vi "main.vi"() -> ()   [LabVIEW 2018]
panel:
  out "开关操作":sgl[](graph)
  out "开关锁止":sgl[](graph)
  out "关开操作":sgl[](graph)
  out "关开锁止":sgl[](graph)
  out "产品名称":string
  in  "产品选择":enum32{"1", "2"}(radio)
  out "ROBOT通讯状态":bool
  out "PLC通讯状态":bool
  out "时刻":string
  in  "参数":bool
  out "F拨钮下上":string
  out "F拨钮上下":string
  out "F拨钮右左":string
  out "F拨钮左右":string
  out "F轮盘开关锁":string
  out "F轮盘开关":string
  out "F轮盘关开锁":string
  out "F轮盘关开":string
  out "LED电流":string
  out "LED电压":string
  out "风门开电压":string
  out "风门闭电压":string
  out "泄漏量结果":string
  out "压力结果":string
  out "漏装3":string
  out "漏装2":string
  out "漏装1":string
  out "风门打开标准":string
  out "风门关闭标准":string
  out "压力标准":string
  out "泄漏量标准":string
  out "LED电压标准":string
  out "LED电流标准":string
  out "拨钮左右标准":string
  out "拨钮右左标准":string
  out "拨钮上下标准":string
  out "拨钮下上标准":string
  out "轮盘关开标准":string
  out "轮盘关开锁止标准":string
  out "轮盘开关标准":string
  out "轮盘开关锁止标准":string
  in  "选项卡控件":T1(tab)
  out "海绵条":bool
  out "小齿轮":bool
  out "连杆":bool
  out "扇齿轮":bool
  out "卡扣左后":bool
  out "卡扣左前":bool
  out "卡扣右后":bool
  out "卡扣右前":bool
  out "金属4":bool
  out "金属3":bool
  out "金属2":bool
  out "金属1":bool
  out "泄漏量":sgl(knob) scale=0.0..30.0
  out "压力":sgl(knob) scale=0.0..800.0
  out "轮盘关开":sgl(graph)
  out "轮盘开关":sgl(graph)
  out "拨钮左右":sgl(graph)
  out "拨钮右左":sgl(graph)
  out "拨钮下上":sgl(graph)
  out "拨钮上下":sgl(graph)
  in  "退出":bool
  out "OK-NG":string
  # "漏装检测"
  # "泄漏检测"
  # "电检"
  # "拨钮操作力（N）"
  # "轮盘操作力矩（Ncm）"
  # "位置"
  # "结果"
  # "标准"
  # "结果"
  # "项目"
  # "标准"
  # "结果"
  # "操作方向"
  # "标准"
  # "结果"
  # "操作方向"
  # "力矩类型"
  # "标准"
  # "结果"
  # "1#位"
  # "风门打开"
  # "左->右"
  # "操作力矩"
  # "关->开"
  # "2#位"
  # "风门关闭"
  # "右->左"
  # "锁止力矩"
  # "3#位"
  # "LED电压"
  # "上->下"
  # "操作力矩"
  # "开->关"
  # "LED电流"
  # "下->上"
  # "锁止力矩"
  # "1#位"
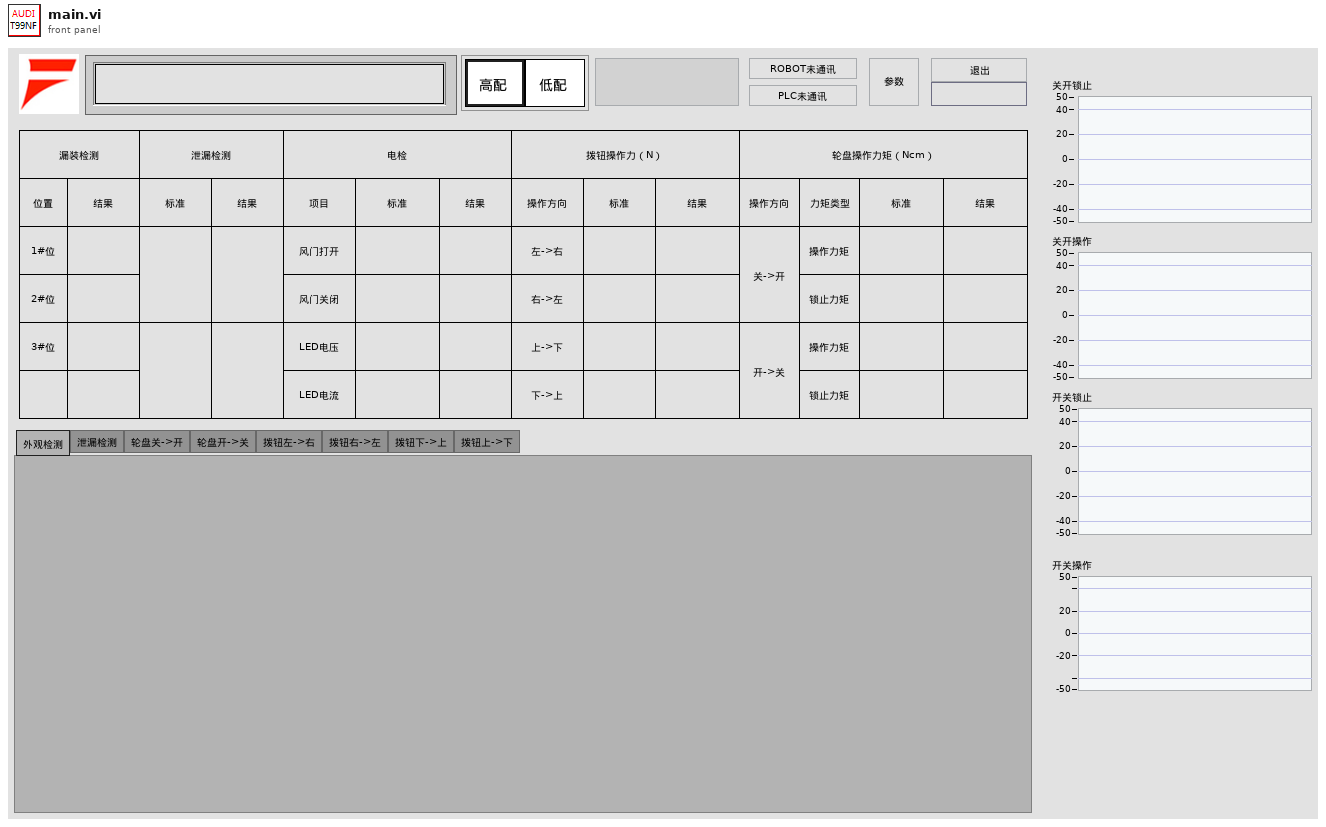
[diagram p1: front panel]
types:
  T1 = enum32{"外观检测", "泄漏检测", "轮盘关->开", "轮盘开->关", "拨钮左->右", "拨钮右->左", "拨钮下->上", "拨钮上->下"}
  T2 = cluster{"压力":string, "泄漏量":string, "风门打开":string, "风门关闭":string, "LED电压":string, "LED电流":string, "拨钮左右":string, "拨钮右左":string, "拨钮上下":string, "拨钮下上":string, "轮盘关开":string, "轮盘关开锁止":string, "轮盘开关":string, "轮盘开关锁止":string}
  T3 = enum16{"Always On", "Always Off", "Off While Running"}
  T4 = cluster{"选择":enum16{"Fx", "Fy", "Fz", "Mx", "My", "Mz"}, "系数":sgl, "上限":sgl, "下限":sgl, "Ymax":dbl, "Ymin":dbl, "点数":dbl, "锁系数x":sgl, "锁上限":sgl, "锁下限":sgl, "锁系数+":sgl, "起点":dbl, "终点":dbl, "锁起点":dbl, "锁终点":dbl}
  T5 = cluster{"选择":enum16{"Fx", "Fy", "Fz", "Mx", "My", "Mz"}, "系数":sgl, "上限":sgl, "下限":sgl, "Ymax":dbl, "Ymin":dbl, "点数":dbl, "起点":dbl, "终点":dbl}
  T6 = cluster{"PLC就绪":bool, "ROBOT就绪":bool, "空动作":bool, "检测NG":bool, "检测结束":bool, "检测开始":bool, "初始化脉冲":bool}
  T7 = cluster{"当前泄漏量":sgl, "稳定泄漏量":sgl, "当前压力":sgl, "稳定压力":sgl, "风门闭电压":sgl, "风门开电压":sgl, "LED电流":sgl, "LED电压":sgl}
  T8 = cluster{"泄漏量":bool, "风门开闭电检":bool, "LED电检":bool, "拍照位1":bool, "拍照位2":bool, "拍照位3":bool, "轮盘关开":bool, "轮盘关开锁":bool, "轮盘开关":bool, "轮盘开关锁":bool, "拨钮左右":bool, "拨钮右左":bool, "拨钮上下":bool, "拨钮下上":bool}
  T9 = cluster{"泄漏量":bool, "风门闭电压":bool, "风门开电压":bool, "LED电压":bool, "LED电流":bool, "拍照1":bool, "拍照2":bool, "拍照3":bool}
  T10 = cluster{"主站IP":u32, "组号":u8, "帧号":u16, "时间戳":u64}
  T11 = cluster{"泄漏量":bool, "轮盘开闭电检":bool, "LED电检":bool, "拍照位1":bool, "拍照位2":bool, "拍照位3":bool, "轮盘关开":bool, "轮盘关开锁":bool, "轮盘开关":bool, "轮盘开关锁":bool, "拨钮左右":bool, "拨钮右左":bool, "拨钮上下":bool, "拨钮下上":bool}
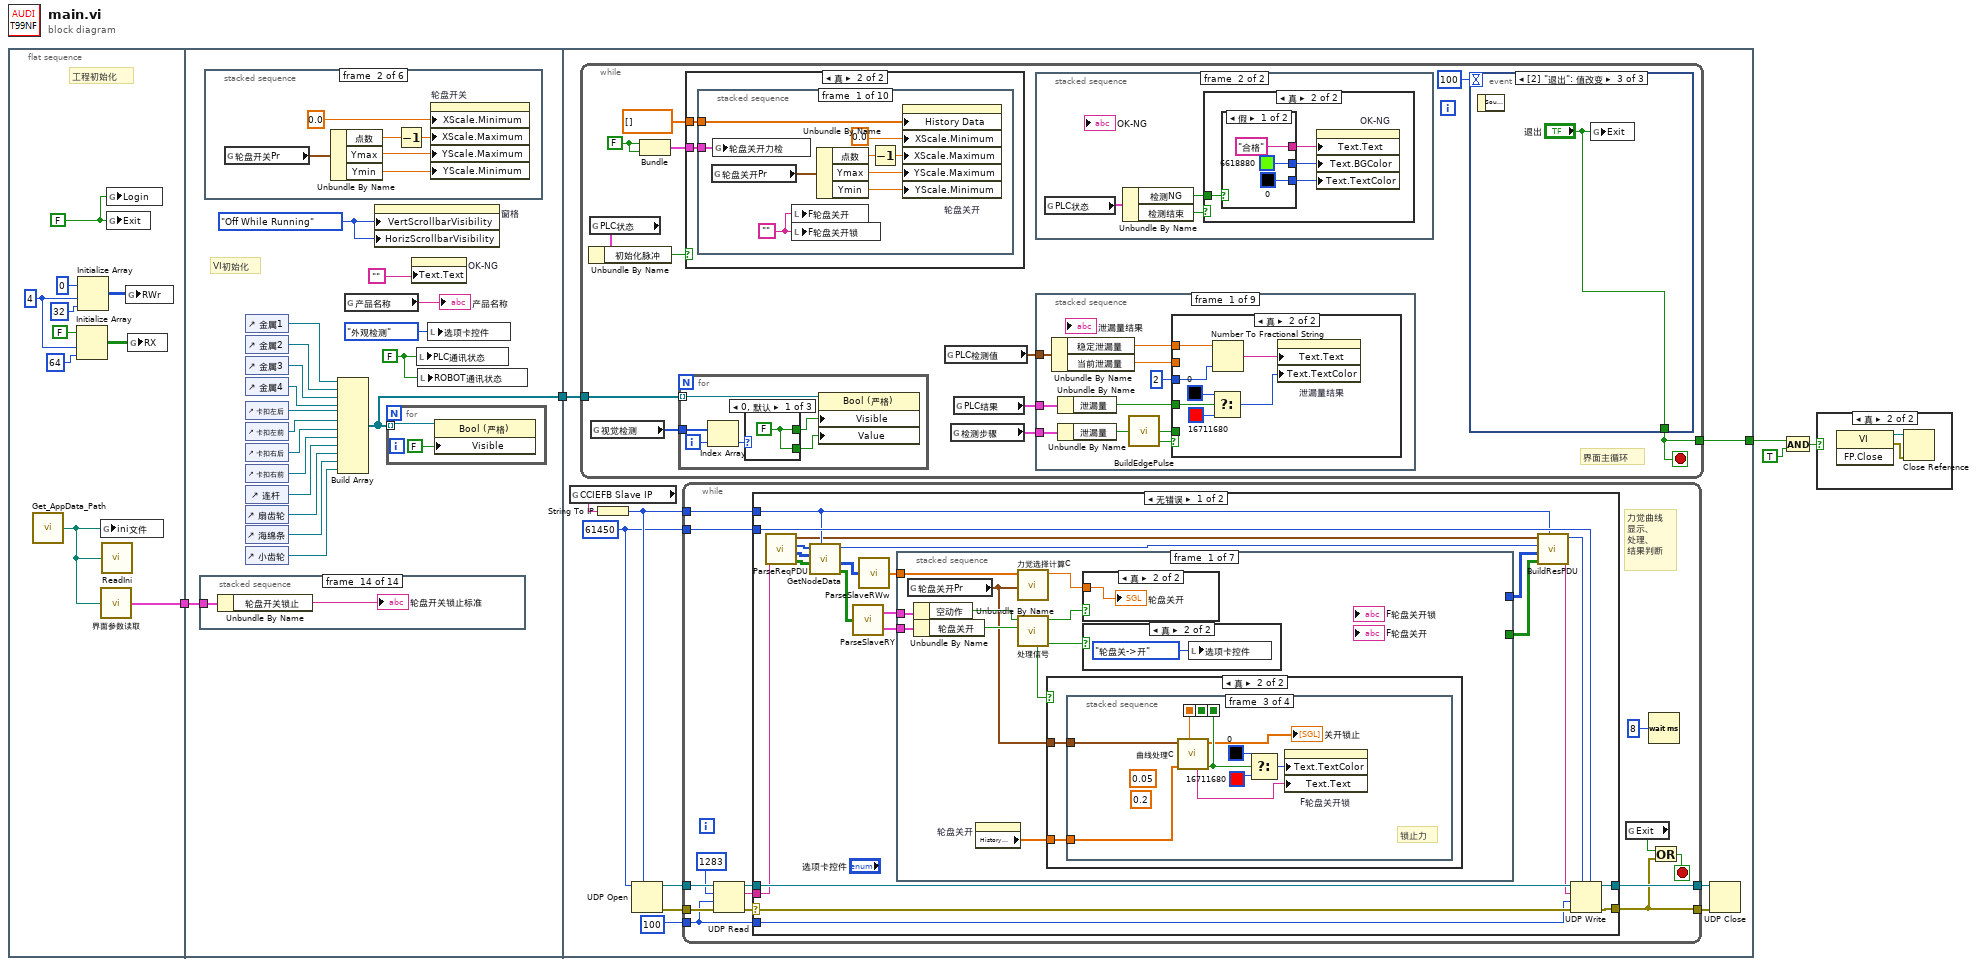
[diagram p0: block diagram]
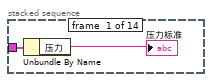
[diagram p2: hidden frame]
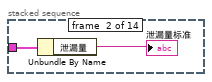
[diagram p3: hidden frame]
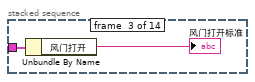
[diagram p4: hidden frame]
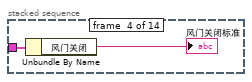
[diagram p5: hidden frame]
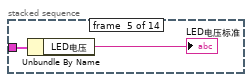
[diagram p6: hidden frame]
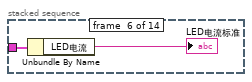
[diagram p7: hidden frame]
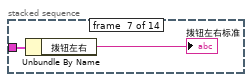
[diagram p8: hidden frame]
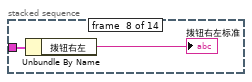
[diagram p9: hidden frame]
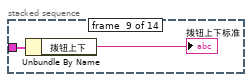
[diagram p10: hidden frame]
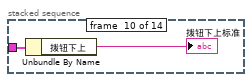
[diagram p11: hidden frame]
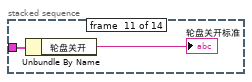
[diagram p12: hidden frame]
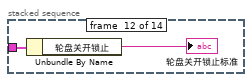
[diagram p13: hidden frame]
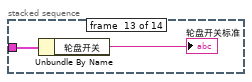
[diagram p14: hidden frame]
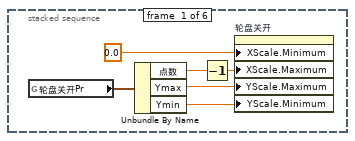
[diagram p15: hidden frame]
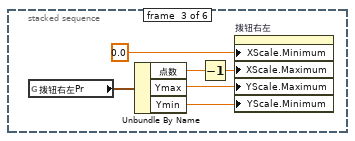
[diagram p16: hidden frame]
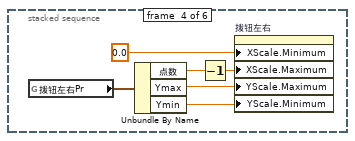
[diagram p17: hidden frame]
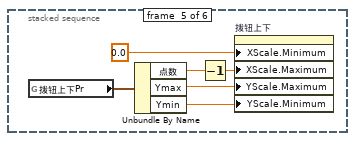
[diagram p18: hidden frame]
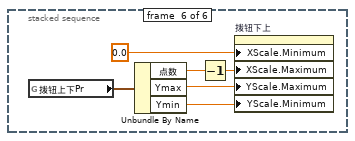
[diagram p19: hidden frame]
diagram:
  n1 = flat-sequence {
    tunnel: [w6] -> w1
    tunnel: [w21] -> w2
    tunnel: w1 -> [w16]
    tunnel: [w110] -> w4
    tunnel: w2 -> [w103]
    frame #0 {
      w11 = 4 ("维数大小")
      w8 = FALSE ("退出")
      # "工程初始化"
      n2 = call "Get_AppData_Path.vi"() -> ("path"=w7:path)  [unwired: 1 in]
      n3 = Initialize Array(FALSE, w11, 64 ("维数大小")) -> (w9:bool[][])
      n4 = Initialize Array(i16 0 ("元素"), w11, 32 ("维数大小")) -> (w14:i16[][])
      n5 = global write "全局 1.vi" "ini文件"(w7) -> ()
      n6 = call "界面参数读取.vi"("路径"=w7) -> ("标准"=w6:T2)
      n7 = call "ReadIni.vi"("configuration file path"=w7) -> ()  [unwired: 1 in]
      n8 = global write "全局 1.vi" "Login"(w8) -> ()
      n9 = global write "全局 1.vi" "Exit"(w8) -> ()
      n10 = global write "全局 1.vi" "RWr"(w14) -> ()
      n11 = global write "全局 1.vi" "RX"(w9) -> ()
    }
    frame #1 {
      w17 = T3."Off While Running" ("垂直滚动条可见")
      w18 = FALSE
      # "VI初始化"
      n12 = stacked-sequence {
        tunnel: w16 -> [w36 w38 w40 w42 w44 w46 w48 w50 w52 w54 w56 w58 w60 w62]
        frame #0 {
          n13 = Unbundle By Name(w36) -> ("压力"=→"压力标准":string)
        }
        frame #1 {
          n14 = Unbundle By Name(w38) -> ("泄漏量"=→"泄漏量标准":string)
        }
        frame #2 {
          n15 = Unbundle By Name(w40) -> ("风门打开"=→"风门打开标准":string)
        }
        frame #3 {
          n16 = Unbundle By Name(w42) -> ("风门关闭"=→"风门关闭标准":string)
        }
        frame #4 {
          n17 = Unbundle By Name(w44) -> ("LED电压"=→"LED电压标准":string)
        }
        frame #5 {
          n18 = Unbundle By Name(w46) -> ("LED电流"=→"LED电流标准":string)
        }
        frame #6 {
          n19 = Unbundle By Name(w48) -> ("拨钮左右"=→"拨钮左右标准":string)
        }
        frame #7 {
          n20 = Unbundle By Name(w50) -> ("拨钮右左"=→"拨钮右左标准":string)
        }
        frame #8 {
          n21 = Unbundle By Name(w52) -> ("拨钮上下"=→"拨钮上下标准":string)
        }
        frame #9 {
          n22 = Unbundle By Name(w54) -> ("拨钮下上"=→"拨钮下上标准":string)
        }
        frame #10 {
          n23 = Unbundle By Name(w56) -> ("轮盘关开"=→"轮盘关开标准":string)
        }
        frame #11 {
          n24 = Unbundle By Name(w58) -> ("轮盘关开锁止"=→"轮盘关开锁止标准":string)
        }
        frame #12 {
          n25 = Unbundle By Name(w60) -> ("轮盘开关"=→"轮盘开关标准":string)
        }
        frame #13 {
          n26 = Unbundle By Name(w62) -> ("轮盘开关锁止"=→"轮盘开关锁止标准":string)
        }
      }
      n27 = stacked-sequence {
        frame #0 {
          n28 = global read "全局 1.vi" "轮盘关开Pr"() -> (w68:T4)
          n29 = Unbundle By Name(w68) -> ("点数"=w64:dbl, "Ymax"=w66:dbl, "Ymin"=w67:dbl)
          n30 = Decrement(x=w64) -> (x-1=w65:dbl)
          n31 = property on="轮盘关开" class="WFChart (严格)"("XScale.Minimum"=0.0, "XScale.Maximum"=w65, "YScale.Maximum"=w66, "YScale.Minimum"=w67) -> ()  [unwired: 2 in, 2 out]
        }
        frame #1 {
          n32 = global read "全局 1.vi" "轮盘开关Pr"() -> (w74:T4)
          n33 = Unbundle By Name(w74) -> ("点数"=w70:dbl, "Ymax"=w72:dbl, "Ymin"=w73:dbl)
          n34 = Decrement(x=w70) -> (x-1=w71:dbl)
          n35 = property on="轮盘开关" class="WFChart (严格)"("XScale.Minimum"=0.0 ("X标尺.范围:最大值"), "XScale.Maximum"=w71, "YScale.Maximum"=w72, "YScale.Minimum"=w73) -> ()  [unwired: 2 in, 2 out]
        }
        frame #2 {
          n36 = global read "全局 1.vi" "拨钮右左Pr"() -> (w80:T5)
          n37 = Unbundle By Name(w80) -> ("点数"=w76:dbl, "Ymax"=w78:dbl, "Ymin"=w79:dbl)
          n38 = Decrement(x=w76) -> (x-1=w77:dbl)
          n39 = property on="拨钮右左" class="WFChart (严格)"("XScale.Minimum"=0.0 ("X标尺.范围:最大值"), "XScale.Maximum"=w77, "YScale.Maximum"=w78, "YScale.Minimum"=w79) -> ()  [unwired: 2 in, 2 out]
        }
        frame #3 {
          n40 = global read "全局 1.vi" "拨钮左右Pr"() -> (w86:T5)
          n41 = Unbundle By Name(w86) -> ("点数"=w82:dbl, "Ymax"=w84:dbl, "Ymin"=w85:dbl)
          n42 = Decrement(x=w82) -> (x-1=w83:dbl)
          n43 = property on="拨钮左右" class="WFChart (严格)"("XScale.Minimum"=0.0 ("X标尺.范围:最大值"), "XScale.Maximum"=w83, "YScale.Maximum"=w84, "YScale.Minimum"=w85) -> ()  [unwired: 2 in, 2 out]
        }
        frame #4 {
          n44 = global read "全局 1.vi" "拨钮上下Pr"() -> (w92:T5)
          n45 = Unbundle By Name(w92) -> ("点数"=w88:dbl, "Ymax"=w90:dbl, "Ymin"=w91:dbl)
          n46 = Decrement(x=w88) -> (x-1=w89:dbl)
          n47 = property on="拨钮上下" class="WFChart (严格)"("XScale.Minimum"=0.0 ("X标尺.范围:最大值"), "XScale.Maximum"=w89, "YScale.Maximum"=w90, "YScale.Minimum"=w91) -> ()  [unwired: 2 in, 2 out]
        }
        frame #5 {
          n48 = global read "全局 1.vi" "拨钮上下Pr"() -> (w98:T5)
          n49 = Unbundle By Name(w98) -> ("点数"=w94:dbl, "Ymax"=w96:dbl, "Ymin"=w97:dbl)
          n50 = Decrement(x=w94) -> (x-1=w95:dbl)
          n51 = property on="拨钮下上" class="WFChart (严格)"("XScale.Minimum"=0.0 ("X标尺.范围:最大值"), "XScale.Maximum"=w95, "YScale.Maximum"=w96, "YScale.Minimum"=w97) -> ()  [unwired: 2 in, 2 out]
        }
      }
      n52 = control-ref of="金属1"() -> (w22:refnum<vi>)
      n53 = control-ref of="金属2"() -> (w23:refnum<vi>)
      n54 = control-ref of="金属3"() -> (w24:refnum<vi>)
      n55 = control-ref of="金属4"() -> (w25:refnum<vi>)
      n56 = control-ref of="卡扣左后"() -> (w26:refnum<vi>)
      n57 = control-ref of="卡扣左前"() -> (w27:refnum<vi>)
      n58 = control-ref of="卡扣右后"() -> (w28:refnum<vi>)
      n59 = control-ref of="卡扣右前"() -> (w29:refnum<vi>)
      n60 = control-ref of="连杆"() -> (w30:refnum<vi>)
      n61 = control-ref of="扇齿轮"() -> (w31:refnum<vi>)
      n62 = control-ref of="海绵条"() -> (w32:refnum<vi>)
      n63 = control-ref of="小齿轮"() -> (w33:refnum<vi>)
      n64 = Build Array(w22, w23, w24, w25, w26, w27, w28, w29, w30, w31, w32, w33) -> (w21:refnum<vi>[])
      n65 = global read "全局 1.vi" "产品名称"() -> (→"产品名称":string)
      n66 = property on="窗格" class="Pane"("VertScrollbarVisibility"=w17, "HorizScrollbarVisibility"=w17) -> ()  [unwired: 2 in, 2 out]
      n67 = for {
        tunnel: w21 -> [w100] mode=indexing
        n68 = property class="Bool (严格)"(reference=w100, "Visible"=FALSE ("可见")) -> ()  [unwired: 1 in, 2 out]
      }
      n69 = property on="OK-NG" class="Str"("Text.Text"="") -> ()  [unwired: 2 in, 2 out]
      n70 = local write "PLC通讯状态"(w18) -> ()
      n71 = local write "ROBOT通讯状态"(w18) -> ()
      n72 = local write "选项卡控件"(T1."外观检测" ("选项卡控件")) -> ()
    }
    frame #2 {
      w104 = u16 61450 ("端口")
      n73 = global read "全局 1.vi" "CCIEFB Slave IP"() -> (w102:string)
      n74 = while {
        tunnel: [w409] -> w110
        tunnel: w103 -> [w407]
        stop <- w409 stop-if-true
        w406 = FALSE
        # "界面主循环"
        n75 = global read "全局 1.vi" "PLC状态"() -> (w404:T6)
        n76 = Unbundle By Name(w404) -> ("初始化脉冲"=w403:bool)
        n77 = global read "全局 1.vi" "视觉检测"() -> (w408:u16[])
        n78 = Bundle(w406, w406) -> (w405:cluster{bool, bool})  [unwired: 1 in]
        n79 = for {
          tunnel: w407 -> [w652] mode=indexing
          tunnel: w408 -> [w655]
          i -> [w654]
          n80 = Index Array(array=w655, index=w654) -> (element=w653:u16)
          n81 = case shown="0, 默认" w653 {
            tunnel: [w656 TRUE TRUE] -> w651
            tunnel: [w656 FALSE TRUE] -> w650
            frame 0, Default {
              w656 = FALSE
            }
            frame 1 {
            }
            frame 2 {
            }
          }
          n82 = property class="Bool (严格)"(reference=w652, "Visible"=w651, "Value"=w650) -> ()  [unwired: 1 in, 2 out]
        }
        n83 = case shown="真" w403 {
          tunnel: w405 -> [_ w590]
          tunnel: sgl[] [] ("历史数据") -> [_ w589]
          frame False {
          }
          frame True {
            n84 = stacked-sequence {
              tunnel: w590 -> [w599 _ w609 _ w619 w628 w637 w646 _ _]
              tunnel: w589 -> [w591 w600 w601 w610 w611 w620 w629 w638 _ _]
              frame #0 {
                w592 = ""
                n85 = global read "全局 1.vi" "轮盘关开Pr"() -> (w597:T4)
                n86 = global write "全局 1.vi" "轮盘关开力检"(w599) -> ()
                n87 = local write "F轮盘关开"(w592) -> ()
                n88 = local write "F轮盘关开锁"(w592) -> ()
                n89 = Unbundle By Name(w597) -> ("点数"=w598:dbl, "Ymax"=w594:dbl, "Ymin"=w593:dbl)
                n90 = Decrement(x=w598) -> (x-1=w596:dbl)
                n91 = property on="轮盘关开" class="WFChart (严格)"("History Data"=w591, "XScale.Minimum"=0.0, "XScale.Maximum"=w596, "YScale.Maximum"=w594, "YScale.Minimum"=w593) -> ()  [unwired: 2 in, 2 out]
              }
              frame #1 {
                n92 = property on="关开锁止" class="WFChart (严格)"("History Data"=w600) -> ()  [unwired: 2 in, 2 out]
                n93 = property on="关开操作" class="WFChart (严格)"("History Data"=w600) -> ()  [unwired: 2 in, 2 out]
              }
              frame #2 {
                w602 = ""
                n94 = global write "全局 1.vi" "轮盘开关力检"(w609) -> ()
                n95 = global read "全局 1.vi" "轮盘开关Pr"() -> (w608:T4)
                n96 = local write "F轮盘开关"(w602) -> ()
                n97 = local write "F轮盘开关锁"(w602) -> ()
                n98 = Unbundle By Name(w608) -> ("点数"=w607:dbl, "Ymax"=w606:dbl, "Ymin"=w605:dbl)
                n99 = Decrement(x=w607) -> (x-1=w604:dbl)
                n100 = property on="轮盘开关" class="WFChart (严格)"("History Data"=w601, "XScale.Minimum"=0.0 ("X标尺.范围:最大值"), "XScale.Maximum"=w604, "YScale.Maximum"=w606, "YScale.Minimum"=w605) -> ()  [unwired: 2 in, 2 out]
              }
              frame #3 {
                n101 = property on="开关锁止" class="WFChart (严格)"("History Data"=w610) -> ()  [unwired: 2 in, 2 out]
                n102 = property on="开关操作" class="WFChart (严格)"("History Data"=w610) -> ()  [unwired: 2 in, 2 out]
              }
              frame #4 {
                n103 = global write "全局 1.vi" "拨钮右左力检"(w619) -> ()
                n104 = global read "全局 1.vi" "拨钮右左Pr"() -> (w618:T5)
                n105 = local write "F拨钮左右"("") -> ()
                n106 = Unbundle By Name(w618) -> ("点数"=w617:dbl, "Ymax"=w614:dbl, "Ymin"=w613:dbl)
                n107 = Decrement(x=w617) -> (x-1=w616:dbl)
                n108 = property on="拨钮右左" class="WFChart (严格)"("History Data"=w611, "XScale.Minimum"=0.0 ("X标尺.范围:最大值"), "XScale.Maximum"=w616, "YScale.Maximum"=w614, "YScale.Minimum"=w613) -> ()  [unwired: 2 in, 2 out]
              }
              frame #5 {
                n109 = global read "全局 1.vi" "拨钮左右Pr"() -> (w627:T5)
                n110 = global write "全局 1.vi" "拨钮左右力检"(w628) -> ()
                n111 = local write "F拨钮右左"("") -> ()
                n112 = Unbundle By Name(w627) -> ("点数"=w626:dbl, "Ymax"=w623:dbl, "Ymin"=w622:dbl)
                n113 = Decrement(x=w626) -> (x-1=w625:dbl)
                n114 = property on="拨钮左右" class="WFChart (严格)"("History Data"=w620, "XScale.Minimum"=0.0 ("X标尺.范围:最大值"), "XScale.Maximum"=w625, "YScale.Maximum"=w623, "YScale.Minimum"=w622) -> ()  [unwired: 2 in, 2 out]
              }
              frame #6 {
                n115 = global read "全局 1.vi" "拨钮上下Pr"() -> (w636:T5)
                n116 = global write "全局 1.vi" "拨钮下上力检"(w637) -> ()
                n117 = local write "F拨钮上下"("") -> ()
                n118 = Unbundle By Name(w636) -> ("点数"=w635:dbl, "Ymax"=w632:dbl, "Ymin"=w631:dbl)
                n119 = Decrement(x=w635) -> (x-1=w634:dbl)
                n120 = property on="拨钮下上" class="WFChart (严格)"("History Data"=w629, "XScale.Minimum"=0.0 ("X标尺.范围:最大值"), "XScale.Maximum"=w634, "YScale.Maximum"=w632, "YScale.Minimum"=w631) -> ()  [unwired: 2 in, 2 out]
              }
              frame #7 {
                n121 = global write "全局 1.vi" "拨钮上下力检"(w646) -> ()
                n122 = global read "全局 1.vi" "拨钮下上Pr"() -> (w645:T5)
                n123 = local write "F拨钮下上"("") -> ()
                n124 = Unbundle By Name(w645) -> ("点数"=w644:dbl, "Ymax"=w641:dbl, "Ymin"=w640:dbl)
                n125 = Decrement(x=w644) -> (x-1=w643:dbl)
                n126 = property on="拨钮上下" class="WFChart (严格)"("History Data"=w638, "XScale.Minimum"=0.0 ("X标尺.范围:最大值"), "XScale.Maximum"=w643, "YScale.Maximum"=w641, "YScale.Minimum"=w640) -> ()  [unwired: 2 in, 2 out]
              }
              frame #8 {
                w647 = ""
                n127 = local write "泄漏量结果"(w647) -> ()
                n128 = local write "风门开电压"(w647) -> ()
                n129 = local write "风门闭电压"(w647) -> ()
                n130 = local write "压力结果"(w647) -> ()
                n131 = local write "LED电压"(w647) -> ()
                n132 = local write "LED电流"(w647) -> ()
                n133 = local write "漏装1"(w647) -> ()
                n134 = local write "漏装2"(w647) -> ()
                n135 = local write "漏装3"(w647) -> ()
              }
              frame #9 {
                n136 = property on="OK-NG" class="Str"("Text.Text"="", "Text.BGColor"=u32 14869218) -> ()  [unwired: 2 in, 2 out]
              }
            }
          }
        }
        n137 = global read "全局 1.vi" "PLC检测值"() -> (w401:T7)
        n138 = global read "全局 1.vi" "检测步骤"() -> (w402:T8)
        n139 = global read "全局 1.vi" "PLC结果"() -> (w400:T9)
        n140 = stacked-sequence {
          frame #0 {
            n141 = global read "全局 1.vi" "PC状态"() -> (w567:cluster{"PLC就绪":bool, "空动作中":bool})
            n142 = Bundle By Name(cluster=w567, "PLC就绪"=TRUE) -> (w565:cluster{"PLC就绪":bool, "空动作中":bool})
            n143 = global read "全局 1.vi" "PLC状态"() -> (w568:T6)
            n144 = To Word Integer(number="产品选择") -> (16bit integer=w575:i16)
            n145 = Format Date/Time String(time format string (%c)="%c\n第%W周 %A" ("时间格式字符串(%c)")) -> (date/time string=→"时刻":string)  [unwired: 2 in]
            n146 = Increment(x=w575) -> (x+1=w573:i16)
            n147 = Unbundle By Name(w568) -> ("PLC就绪"=→"PLC通讯状态":bool, "ROBOT就绪"=→"ROBOT通讯状态":bool)
            n148 = global write "全局 1.vi" "PC状态"(w565) -> ()
            n149 = global write "全局 1.vi" "高低配"(w573) -> ()
          }
          frame #1 {
            n150 = global read "全局 1.vi" "PLC状态"() -> (w578:T6)
            n151 = Unbundle By Name(w578) -> ("检测NG"=w576:bool, "检测结束"=w577:bool)
            n152 = case shown="真" w577 {
              tunnel: w576 -> [_ w582]
              frame False {
              }
              frame True {
                n153 = case shown="假" w582 {
                  tunnel: ["合格" "不合格"] -> w581
                  tunnel: [u32 6618880 u32 16711680] -> w580
                  tunnel: [u32 0 u32 16448250] -> w579
                  frame False {
                  }
                  frame True {
                  }
                }
                n154 = property on="OK-NG" class="Str"("Text.Text"=w581, "Text.BGColor"=w580, "Text.TextColor"=w579) -> ()  [unwired: 2 in, 2 out]
              }
            }
          }
        }
        n155 = stacked-sequence {
          tunnel: w402 -> [w420 w444 w467 w483 w499 w515 w527 w541 w555]
          tunnel: w401 -> [w417 w441 w464 w480 w496 w512 _ _ _]
          tunnel: w400 -> [w413 w437 w461 w477 w493 w509 w524 w538 w552]
          frame #0 {
            n156 = Unbundle By Name(w417) -> ("稳定泄漏量"=w415:sgl, "当前泄漏量"=w416:sgl)
            n157 = Unbundle By Name(w413) -> ("泄漏量"=w412:bool)
            n158 = Unbundle By Name(w420) -> ("泄漏量"=w419:bool)
            n159 = call "BuildEdgePulse.vi"("输入"=w419) -> ("下降沿"=w418:bool, "输出"=w414:bool)  [unwired: 2 in, 1 out]
            n160 = case shown="真" w418 {
              tunnel: w416 -> [w423 _]
              tunnel: w415 -> [_ w433]
              tunnel: w414 -> [w422 _]
              tunnel: w412 -> [_ w432]
              tunnel: i16 2 ("精度(6)") -> [w421 w428]
              frame False {
                n161 = case shown="真" w422 {
                  tunnel: w423 -> [_ w425]
                  tunnel: w421 -> [_ w424]
                  frame False {
                  }
                  frame True {
                    n162 = Number To Fractional String(number=w425, precision (6)=w424) -> (F-format string=w427:string)  [unwired: 2 in]
                    n163 = property on="泄漏量结果" class="Str"("Text.Text"=w427, "Text.TextColor"=u32 0) -> ()  [unwired: 2 in, 2 out]
                    "泄漏量" <- w425
                  }
                }
              }
              frame True {
                n164 = Select(t=u32 0, s=w432, f=u32 16711680) -> (s? t:f=w429:u32)
                n165 = Number To Fractional String(number=w433, precision (6)=w428) -> (F-format string=w434:string)  [unwired: 2 in]
                n166 = property on="泄漏量结果" class="Str"("Text.Text"=w434, "Text.TextColor"=w429) -> ()  [unwired: 2 in, 2 out]
              }
            }
          }
          frame #1 {
            n167 = Unbundle By Name(w441) -> ("稳定压力"=w439:sgl, "当前压力"=w440:sgl)
            n168 = Unbundle By Name(w437) -> ("泄漏量"=w436:bool)
            n169 = Unbundle By Name(w444) -> ("泄漏量"=w443:bool)
            n170 = call "BuildEdgePulse.vi"("输入"=w443) -> ("下降沿"=w442:bool, "输出"=w438:bool)  [unwired: 2 in, 1 out]
            n171 = case shown="假" w442 {
              tunnel: w440 -> [w447 _]
              tunnel: w439 -> [_ w457]
              tunnel: w438 -> [w446 _]
              tunnel: w436 -> [_ w456]
              tunnel: i16 1 ("精度(6)") -> [w445 w452]
              frame False {
                n172 = case shown="真" w446 {
                  tunnel: w447 -> [_ w449]
                  tunnel: w445 -> [_ w448]
                  frame False {
                  }
                  frame True {
                    n173 = Number To Fractional String(number=w449, precision (6)=w448) -> (F-format string=w451:string)  [unwired: 2 in]
                    n174 = property on="压力结果" class="Str"("Text.Text"=w451, "Text.TextColor"=u32 0) -> ()  [unwired: 2 in, 2 out]
                    "压力" <- w449
                  }
                }
              }
              frame True {
                n175 = Select(t=u32 0, s=w456, f=u32 16711680) -> (s? t:f=w453:u32)
                n176 = Number To Fractional String(number=w457, precision (6)=w452) -> (F-format string=w458:string)  [unwired: 2 in]
                n177 = property on="压力结果" class="Str"("Text.Text"=w458, "Text.TextColor"=w453) -> ()  [unwired: 2 in, 2 out]
              }
            }
          }
          frame #2 {
            n178 = Unbundle By Name(w467) -> ("风门开闭电检"=w466:bool)
            n179 = Unbundle By Name(w461) -> ("风门开电压"=w460:bool)
            n180 = Unbundle By Name(w464) -> ("风门开电压"=w463:sgl)
            n181 = call "BuildEdgePulse.vi"("输入"=w466) -> ("下降沿"=w465:bool, "输出"=w462:bool)  [unwired: 2 in, 1 out]
            n182 = case shown="真" w465 {
              tunnel: w463 -> [_ w474]
              tunnel: w462 -> [_ _]
              tunnel: w460 -> [_ w473]
              tunnel: i16 2 ("精度(6)") -> [_ w469]
              frame False {
              }
              frame True {
                n183 = Number To Fractional String(number=w474, precision (6)=w469) -> (F-format string=→"风门开电压":string)  [unwired: 2 in]
                n184 = Select(t=u32 0, s=w473, f=u32 16711680) -> (s? t:f=w470:u32)
                n185 = property on="风门开电压" class="Str"("Text.TextColor"=w470) -> ()  [unwired: 2 in, 2 out]
              }
            }
          }
          frame #3 {
            n186 = Unbundle By Name(w483) -> ("风门开闭电检"=w482:bool)
            n187 = Unbundle By Name(w477) -> ("风门闭电压"=w476:bool)
            n188 = Unbundle By Name(w480) -> ("风门闭电压"=w479:sgl)
            n189 = call "BuildEdgePulse.vi"("输入"=w482) -> ("下降沿"=w481:bool, "输出"=w478:bool)  [unwired: 2 in, 1 out]
            n190 = case shown="真" w481 {
              tunnel: w479 -> [_ w490]
              tunnel: w478 -> [_ _]
              tunnel: w476 -> [_ w489]
              tunnel: i16 2 ("精度(6)") -> [_ w485]
              frame False {
              }
              frame True {
                n191 = Number To Fractional String(number=w490, precision (6)=w485) -> (F-format string=→"风门闭电压":string)  [unwired: 2 in]
                n192 = Select(t=u32 0, s=w489, f=u32 16711680) -> (s? t:f=w486:u32)
                n193 = property on="风门闭电压" class="Str"("Text.TextColor"=w486) -> ()  [unwired: 2 in, 2 out]
              }
            }
          }
          frame #4 {
            n194 = Unbundle By Name(w493) -> ("LED电压"=w492:bool)
            n195 = Unbundle By Name(w499) -> ("LED电检"=w498:bool)
            n196 = Unbundle By Name(w496) -> ("LED电压"=w495:sgl)
            n197 = call "BuildEdgePulse.vi"("输入"=w498) -> ("下降沿"=w497:bool, "输出"=w494:bool)  [unwired: 2 in, 1 out]
            n198 = case shown="真" w497 {
              tunnel: w495 -> [_ w506]
              tunnel: w494 -> [_ _]
              tunnel: w492 -> [_ w505]
              tunnel: i16 2 ("精度(6)") -> [_ w501]
              frame False {
              }
              frame True {
                n199 = Number To Fractional String(number=w506, precision (6)=w501) -> (F-format string=→"LED电压":string)  [unwired: 2 in]
                n200 = Select(t=u32 0, s=w505, f=u32 16711680) -> (s? t:f=w502:u32)
                n201 = property on="LED电压" class="Str"("Text.TextColor"=w502) -> ()  [unwired: 2 in, 2 out]
              }
            }
          }
          frame #5 {
            n202 = Unbundle By Name(w509) -> ("LED电流"=w508:bool)
            n203 = Unbundle By Name(w515) -> ("LED电检"=w514:bool)
            n204 = Unbundle By Name(w512) -> ("LED电流"=w511:sgl)
            n205 = call "BuildEdgePulse.vi"("输入"=w514) -> ("下降沿"=w513:bool, "输出"=w510:bool)  [unwired: 2 in, 1 out]
            n206 = case shown="真" w513 {
              tunnel: w511 -> [_ w522]
              tunnel: w510 -> [_ _]
              tunnel: w508 -> [_ w521]
              tunnel: i16 2 ("精度(6)") -> [_ w517]
              frame False {
              }
              frame True {
                n207 = Number To Fractional String(number=w522, precision (6)=w517) -> (F-format string=→"LED电流":string)  [unwired: 2 in]
                n208 = Select(t=u32 0, s=w521, f=u32 16711680) -> (s? t:f=w518:u32)
                n209 = property on="LED电流" class="Str"("Text.TextColor"=w518) -> ()  [unwired: 2 in, 2 out]
              }
            }
          }
          frame #6 {
            n210 = Unbundle By Name(w527) -> ("拍照位1"=w526:bool)
            n211 = Unbundle By Name(w524) -> ("拍照1"=w523:bool)
            n212 = call "BuildEdgePulse.vi"("输入"=w526) -> ("下降沿"=w525:bool, "上升沿"=w528:bool)  [unwired: 2 in, 1 out]
            n213 = case shown="真" w528 {
              frame False {
              }
              frame True {
                n214 = local write "选项卡控件"(T1."外观检测" ("选项卡控件")) -> ()
              }
            }
            n215 = case shown="真" w525 {
              tunnel: w523 -> [_ w531]
              frame False {
              }
              frame True {
                n216 = case shown="假" w531 {
                  tunnel: ["NG" ("文本.文本") "OK" ("文本.文本")] -> w530
                  tunnel: [u32 16711680 u32 0] -> w529
                  frame False {
                  }
                  frame True {
                  }
                }
                n217 = property on="漏装1" class="Str"("Text.Text"=w530, "Text.TextColor"=w529) -> ()  [unwired: 2 in, 2 out]
              }
            }
          }
          frame #7 {
            n218 = Unbundle By Name(w541) -> ("拍照位2"=w540:bool)
            n219 = Unbundle By Name(w538) -> ("拍照2"=w537:bool)
            n220 = call "BuildEdgePulse.vi"("输入"=w540) -> ("下降沿"=w539:bool, "上升沿"=w542:bool)  [unwired: 2 in, 1 out]
            n221 = case shown="真" w542 {
              frame False {
              }
              frame True {
                n222 = local write "选项卡控件"(T1."外观检测" ("选项卡控件")) -> ()
              }
            }
            n223 = case shown="真" w539 {
              tunnel: w537 -> [_ w545]
              frame False {
              }
              frame True {
                n224 = case shown="假" w545 {
                  tunnel: ["NG" ("文本.文本") "OK" ("文本.文本")] -> w544
                  tunnel: [u32 16711680 u32 0] -> w543
                  frame False {
                  }
                  frame True {
                  }
                }
                n225 = property on="漏装2" class="Str"("Text.Text"=w544, "Text.TextColor"=w543) -> ()  [unwired: 2 in, 2 out]
              }
            }
          }
          frame #8 {
            n226 = Unbundle By Name(w555) -> ("拍照位3"=w554:bool)
            n227 = Unbundle By Name(w552) -> ("拍照3"=w551:bool)
            n228 = call "BuildEdgePulse.vi"("输入"=w554) -> ("下降沿"=w553:bool, "上升沿"=w556:bool)  [unwired: 2 in, 1 out]
            n229 = case shown="真" w556 {
              frame False {
              }
              frame True {
                n230 = local write "选项卡控件"(T1."外观检测" ("选项卡控件")) -> ()
              }
            }
            n231 = case shown="真" w553 {
              tunnel: w551 -> [_ w559]
              frame False {
              }
              frame True {
                n232 = case shown="假" w559 {
                  tunnel: ["NG" ("文本.文本") "OK" ("文本.文本")] -> w558
                  tunnel: [u32 16711680 u32 0] -> w557
                  frame False {
                  }
                  frame True {
                  }
                }
                n233 = property on="漏装3" class="Str"("Text.Text"=w558, "Text.TextColor"=w557) -> ()  [unwired: 2 in, 2 out]
              }
            }
          }
        }
        n234 = event shown="[2] \"退出\": 值改变" {
          selector: _ -> [_ _ _]
          dyn-events: _ -> [_ _ _]
          timeout: 100 ("等待时间（毫秒）") -> [_ _ _]
          tunnel: [_ _ "退出"] -> w409
          event Timeout {
            n235 = event-data() -> ()  [unwired: 1 in, 1 out]
          }
          event "参数": Mouse Up {
            w664 = FALSE ("结束前等待")
            n236 = event-data() -> ()  [unwired: 1 in, 1 out]
            n237 = vi-ref "参数.vi"() -> (w665:refnum<vi>)
            n238 = invoke class="VI" method="Run VI"(reference=w665, "Wait until done"=w664, "Auto Dispose Ref"=w664) -> (reference out=w663:refnum<vi>)  [unwired: 2 in, 4 out]
            n239 = invoke class="VI" method="FP.Open"(reference=w663) -> (reference out=w661:refnum<vi>, error out=w662:errorcluster)  [unwired: 4 in, 3 out]
            n240 = Close Reference(reference=w661, error in (no error)=w662) -> ()  [unwired: 1 out]
          }
          event "退出": Value Change {
            n241 = event-data() -> ()  [unwired: 1 in, 1 out]
            n242 = global write "全局 1.vi" "Exit"("退出") -> ()
          }
        }
      }
      n243 = String To IP(1:w102) -> (0:w105:u32)
      n244 = UDP Open(7:w105, 11:w104) -> (port=w109:refnum<k16>, 0:w107:errorcluster)  [unwired: 3 in, 1 out]
      n245 = while {
        tunnel: w109 -> [w124]
        tunnel: [w115] -> w108
        tunnel: w107 -> [w123]
        tunnel: [w113] -> w106
        tunnel: w105 -> [w117]
        tunnel: w104 -> [w116]
        tunnel: 100 ("超时毫秒(25000)") -> [w111]
        stop <- w120 stop-if-true
        # "力觉曲线\n显示、\n处理、\n结果判断"
        n246 = UDP Read(connection ID=w124, max size (548)=1283 ("最大值(548)"), timeout ms (25000)=w111, 8:w123) -> (data out=w121:string, error out=w122:errorcluster, 3:w118:refnum<k16>)  [unwired: 2 out]
        n247 = case shown="无错误" w122 {
          selector: w122 -> [w146 w395]
          tunnel: w121 -> [w141 _]
          tunnel: [w145 w394] -> w113
          tunnel: w118 -> [w144 w393]
          tunnel: w117 -> [w138 _]
          tunnel: w116 -> [w142 _]
          tunnel: [w143 w393] -> w115
          tunnel: w111 -> [w133 _]
          frame No Error {
            n248 = call "ParseReqPDU.vi"("数据in"=w141) -> ("All RY"=w134:bool[][], "All RWw"=w135:u16[][], "从站IP组"=w137:u32[], "主站信息"=w132:T10)  [unwired: 7 in]
            n249 = call "GetNodeData.vi"("指定从站IP"=w138, "All RY in"=w134, "All RWw in"=w135, "从站IP组"=w137) -> ("Node RY"=w129:bool[][], "Node RWw"=w130:u16[][], "占用站数"=w136:i32)  [unwired: 5 in]
            n250 = call "ParseSlaveRY.vi"("RY"=w129) -> ("PLC状态"=w128:T6, "检测步骤"=w127:T11)
            n251 = call "ParseSlaveRWw.vi"("Node RWw"=w130) -> ("力觉力"=w131:sgl[])
            n252 = stacked-sequence {
              tunnel: w131 -> [w155 w203 w253 w290 w327 w364 _]
              tunnel: w128 -> [w157 w205 w252 w289 w326 w363 _]
              tunnel: w127 -> [w156 w204 w251 w288 w325 w362 _]
              tunnel: [_ _ _ _ _ _ w392] -> w126
              tunnel: [_ _ _ _ _ _ w391] -> w125
              frame #0 {
                n253 = global read "全局 1.vi" "轮盘关开Pr"() -> (w147:T4)
                n254 = Unbundle By Name(w157) -> ("空动作"=w152:bool)
                n255 = Unbundle By Name(w156) -> ("轮盘关开"=w153:bool)
                n256 = property on="轮盘关开" class="WFChart (严格)"() -> ("History Data"=w154:sgl[])  [unwired: 2 in, 2 out]
                n257 = call "力觉选择计算C.vi"("力参数C"=w147, "力"=w155) -> ("曲线"=w150:sgl)  [unwired: 8 in, 1 out]
                n258 = call "处理信号.vi"("动作"=w153, "空动作"=w152) -> ("切换"=w149:bool, "显示曲线"=w151:bool, "判断"=w148:bool)  [unwired: 7 in]
                n259 = case shown="真" w148 {
                  tunnel: w147 -> [_ w161]
                  tunnel: w154 -> [_ w160]
                  frame False {
                  }
                  frame True {
                    n260 = stacked-sequence {
                      seq-local: [_ w175 _ _] -> [_ _ _ w189]
                      seq-local: [_ w167 _ _] -> [_ _ w185 _]
                      seq-local: [_ _ w183 _] -> [_ _ _ w190]
                      tunnel: w161 -> [_ w173 w181 _]
                      tunnel: w160 -> [w162 w174 w180 _]
                      frame #0 {
                        # "显示曲线"
                        n261 = Array Size(array=w162) -> (size(s)=w165:i32)
                        n262 = Decrement(x=w165) -> (x-1=w164:i32)
                        n263 = To Double Precision Float(number=w164) -> (double precision float=w163:dbl)
                        n264 = property on="轮盘关开" class="WFChart (严格)"("History Data"=w162, "XScale.Maximum"=w163, "XScale.Minimum"=0.0 ("X标尺.范围:最小值")) -> ()  [unwired: 2 in, 2 out]
                      }
                      frame #1 {
                        # "操作力"
                        n265 = Unbundle By Name(w173) -> ("上限"=w172:sgl, "下限"=w171:sgl, "起点"=w169:dbl, "终点"=w168:dbl)
                        n266 = call "曲线处理.vi"("上限"=w172, "下限"=w171, "起点"=w169, "终点"=w168, "历史数据"=w174) -> ("值"=w167:sgl, "值显示"=w176:string, "曲线数组"=→"关开操作":sgl[], "范围内?"=w175:bool)  [unwired: 2 in]
                        n267 = Select(t=u32 0, s=w175, f=u32 16711680) -> (s? t:f=w177:u32)
                        n268 = property on="F轮盘关开" class="Str"("Text.TextColor"=w177, "Text.Text"=w176) -> ()  [unwired: 2 in, 2 out]
                      }
                      frame #2 {
                        (unwired) 0.05 ("终点(0%)")
                        (unwired) 0.2 ("终点(0%)")
                        # "锁止力"
                        n269 = call "曲线处理C.vi"("基值"=w185, "历史数据"=w180, "力觉参数C"=w181) -> ("范围内?"=w183:bool, "曲线数组"=→"关开锁止":sgl[], "值显示"=w186:string)  [unwired: 6 in]
                        n270 = Select(t=u32 0, s=w183, f=u32 16711680) -> (s? t:f=w187:u32)
                        n271 = property on="F轮盘关开锁" class="Str"("Text.TextColor"=w187, "Text.Text"=w186) -> ()  [unwired: 2 in, 2 out]
                      }
                      frame #3 {
                        n272 = Not And(1:w189, 2:w190) -> (0:w191:bool)
                        n273 = global read "全局 1.vi" "轮盘关开力检"() -> (w192:cluster{"判断完成":bool, "不合格?":bool})
                        n274 = Bundle By Name(cluster=w192, "判断完成"=TRUE, "不合格?"=w191) -> (w194:cluster{"判断完成":bool, "不合格?":bool})
                        n275 = global write "全局 1.vi" "轮盘关开力检"(w194) -> ()
                      }
                    }
                  }
                }
                n276 = case shown="真" w151 {
                  tunnel: w150 -> [_ w159]
                  frame False {
                  }
                  frame True {
                    "轮盘关开" <- w159
                  }
                }
                n277 = case shown="真" w149 {
                  frame False {
                  }
                  frame True {
                    n278 = local write "选项卡控件"(T1."轮盘关->开" ("选项卡控件")) -> ()
                  }
                }
              }
              frame #1 {
                n279 = global read "全局 1.vi" "轮盘开关Pr"() -> (w195:T4)
                n280 = Unbundle By Name(w205) -> ("空动作"=w200:bool)
                n281 = Unbundle By Name(w204) -> ("轮盘开关"=w201:bool)
                n282 = property on="轮盘开关" class="WFChart (严格)"() -> ("History Data"=w202:sgl[])  [unwired: 2 in, 2 out]
                n283 = call "处理信号.vi"("动作"=w201, "空动作"=w200) -> ("切换"=w197:bool, "显示曲线"=w199:bool, "判断"=w196:bool)  [unwired: 7 in]
                n284 = call "力觉选择计算C.vi"("力参数C"=w195, "力"=w203) -> ("曲线"=w198:sgl)  [unwired: 8 in, 1 out]
                n285 = case shown="真" w196 {
                  tunnel: w195 -> [_ w209]
                  tunnel: w202 -> [_ w208]
                  frame False {
                  }
                  frame True {
                    n286 = stacked-sequence {
                      seq-local: [_ w223 _ _] -> [_ _ _ w237]
                      seq-local: [_ w217 _ _] -> [_ _ w233 _]
                      seq-local: [_ _ w231 _] -> [_ _ _ w238]
                      tunnel: w209 -> [_ w221 w229 _]
                      tunnel: w208 -> [w210 w222 w228 _]
                      frame #0 {
                        # "显示曲线"
                        n287 = Array Size(array=w210) -> (size(s)=w213:i32)
                        n288 = Decrement(x=w213) -> (x-1=w212:i32)
                        n289 = To Double Precision Float(number=w212) -> (double precision float=w211:dbl)
                        n290 = property on="轮盘开关" class="WFChart (严格)"("History Data"=w210, "XScale.Maximum"=w211, "XScale.Minimum"=0.0 ("X标尺.范围:最小值")) -> ()  [unwired: 2 in, 2 out]
                      }
                      frame #1 {
                        # "操作力"
                        n291 = Unbundle By Name(w221) -> ("上限"=w220:sgl, "下限"=w219:sgl, "起点"=w216:dbl, "终点"=w215:dbl)
                        n292 = call "曲线处理.vi"("上限"=w220, "下限"=w219, "起点"=w216, "终点"=w215, "历史数据"=w222) -> ("值"=w217:sgl, "值显示"=w224:string, "曲线数组"=→"开关操作":sgl[], "范围内?"=w223:bool)  [unwired: 2 in]
                        n293 = Select(t=u32 0, s=w223, f=u32 16711680) -> (s? t:f=w225:u32)
                        n294 = property on="F轮盘开关" class="Str"("Text.TextColor"=w225, "Text.Text"=w224) -> ()  [unwired: 2 in, 2 out]
                      }
                      frame #2 {
                        (unwired) 0.05 ("终点(0%)")
                        (unwired) 0.2 ("终点(0%)")
                        # "锁止力"
                        n295 = call "曲线处理C.vi"("基值"=w233, "历史数据"=w228, "力觉参数C"=w229) -> ("范围内?"=w231:bool, "曲线数组"=→"开关锁止":sgl[], "值显示"=w234:string)  [unwired: 6 in]
                        n296 = Select(t=u32 0, s=w231, f=u32 16711680) -> (s? t:f=w235:u32)
                        n297 = property on="F轮盘开关锁" class="Str"("Text.TextColor"=w235, "Text.Text"=w234) -> ()  [unwired: 2 in, 2 out]
                      }
                      frame #3 {
                        n298 = Not And(1:w237, 2:w238) -> (0:w239:bool)
                        n299 = global read "全局 1.vi" "轮盘开关力检"() -> (w240:cluster{"判断完成":bool, "不合格?":bool})
                        n300 = Bundle By Name(cluster=w240, "判断完成"=TRUE, "不合格?"=w239) -> (w242:cluster{"判断完成":bool, "不合格?":bool})
                        n301 = global write "全局 1.vi" "轮盘开关力检"(w242) -> ()
                      }
                    }
                  }
                }
                n302 = case shown="真" w199 {
                  tunnel: w198 -> [_ w207]
                  frame False {
                  }
                  frame True {
                    "轮盘开关" <- w207
                  }
                }
                n303 = case shown="真" w197 {
                  frame False {
                  }
                  frame True {
                    n304 = local write "选项卡控件"(T1."轮盘开->关" ("选项卡控件")) -> ()
                  }
                }
              }
              frame #2 {
                n305 = global read "全局 1.vi" "拨钮左右Pr"() -> (w243:T5)
                n306 = Unbundle By Name(w252) -> ("空动作"=w247:bool)
                n307 = Unbundle By Name(w251) -> ("拨钮左右"=w248:bool)
                n308 = property on="拨钮左右" class="WFChart (严格)"() -> ("History Data"=w249:sgl[])  [unwired: 2 in, 2 out]
                n309 = call "处理信号.vi"("动作"=w248, "空动作"=w247) -> ("切换"=w245:bool, "显示曲线"=w246:bool, "判断"=w244:bool)  [unwired: 7 in]
                n310 = call "显示曲线.vi"("力觉参数"=w243, "力数组"=w253) -> ("力值"=w250:sgl)  [unwired: 1 in]
                n311 = case shown="真" w244 {
                  tunnel: w249 -> [_ w260]
                  tunnel: w243 -> [_ w259]
                  frame False {
                  }
                  frame True {
                    n312 = Unbundle By Name(w259) -> ("上限"=w257:sgl, "下限"=w258:sgl, "起点"=w256:dbl, "终点"=w255:dbl)
                    n313 = call "曲线处理.vi"("上限"=w257, "下限"=w258, "起点"=w256, "终点"=w255, "历史数据"=w260) -> ("值显示"=w261:string, "曲线数组"=w263:sgl[], "范围内?"=w262:bool)  [unwired: 2 in, 1 out]
                    n314 = stacked-sequence {
                      tunnel: w263 -> [w268 _ _]
                      tunnel: w262 -> [_ w273 w278]
                      tunnel: w261 -> [_ _ w274]
                      frame #0 {
                        n315 = Array Size(array=w268) -> (size(s)=w265:i32)
                        n316 = Decrement(x=w265) -> (x-1=w264:i32)
                        n317 = To Double Precision Float(number=w264) -> (double precision float=w267:dbl)
                        n318 = property on="拨钮左右" class="WFChart (严格)"("History Data"=w268, "XScale.Maximum"=w267, "XScale.Minimum"=0.0 ("X标尺.范围:最小值")) -> ()  [unwired: 2 in, 2 out]
                      }
                      frame #1 {
                        n319 = global read "全局 1.vi" "拨钮左右力检"() -> (w269:cluster{"判断完成":bool, "不合格?":bool})
                        n320 = Not(x=w273) -> (.not. x?=w271:bool)
                        n321 = Bundle By Name(cluster=w269, "判断完成"=TRUE, "不合格?"=w271) -> (w272:cluster{"判断完成":bool, "不合格?":bool})
                        n322 = global write "全局 1.vi" "拨钮左右力检"(w272) -> ()
                      }
                      frame #2 {
                        n323 = Select(t=u32 0, s=w278, f=u32 16711680) -> (s? t:f=w275:u32)
                        n324 = property on="F拨钮左右" class="Str"("Text.TextColor"=w275, "Text.Text"=w274) -> ()  [unwired: 2 in, 2 out]
                      }
                    }
                  }
                }
                n325 = case shown="真" w246 {
                  tunnel: w250 -> [_ w279]
                  frame False {
                  }
                  frame True {
                    "拨钮左右" <- w279
                  }
                }
                n326 = case shown="真" w245 {
                  frame False {
                  }
                  frame True {
                    n327 = local write "选项卡控件"(T1."拨钮左->右" ("选项卡控件")) -> ()
                  }
                }
              }
              frame #3 {
                n328 = Unbundle By Name(w289) -> ("空动作"=w284:bool)
                n329 = Unbundle By Name(w288) -> ("拨钮右左"=w285:bool)
                n330 = global read "全局 1.vi" "拨钮右左Pr"() -> (w280:T5)
                n331 = property on="拨钮右左" class="WFChart (严格)"() -> ("History Data"=w286:sgl[])  [unwired: 2 in, 2 out]
                n332 = call "显示曲线.vi"("力觉参数"=w280, "力数组"=w290) -> ("力值"=w287:sgl)  [unwired: 1 in]
                n333 = call "处理信号.vi"("动作"=w285, "空动作"=w284) -> ("切换"=w282:bool, "显示曲线"=w283:bool, "判断"=w281:bool)  [unwired: 7 in]
                n334 = case shown="真" w281 {
                  tunnel: w286 -> [_ w296]
                  tunnel: w280 -> [_ w293]
                  frame False {
                  }
                  frame True {
                    n335 = Unbundle By Name(w293) -> ("上限"=w294:sgl, "下限"=w295:sgl, "起点"=w292:dbl, "终点"=w291:dbl)
                    n336 = call "曲线处理.vi"("上限"=w294, "下限"=w295, "起点"=w292, "终点"=w291, "历史数据"=w296) -> ("值显示"=w298:string, "曲线数组"=w299:sgl[], "范围内?"=w297:bool)  [unwired: 2 in, 1 out]
                    n337 = stacked-sequence {
                      tunnel: w299 -> [w304 _ _]
                      tunnel: w298 -> [_ _ w310]
                      tunnel: w297 -> [_ w307 w312]
                      frame #0 {
                        n338 = Array Size(array=w304) -> (size(s)=w303:i32)
                        n339 = To Double Precision Float(number=w303) -> (double precision float=w302:dbl)
                        n340 = Decrement(x=w302) -> (x-1=w301:dbl)
                        n341 = property on="拨钮右左" class="WFChart (严格)"("History Data"=w304, "XScale.Maximum"=w301, "XScale.Minimum"=0.0 ("X标尺.范围:最小值")) -> ()  [unwired: 2 in, 2 out]
                      }
                      frame #1 {
                        n342 = global read "全局 1.vi" "拨钮右左力检"() -> (w305:cluster{"判断完成":bool, "不合格?":bool})
                        n343 = Not(x=w307) -> (.not. x?=w309:bool)
                        n344 = Bundle By Name(cluster=w305, "判断完成"=TRUE, "不合格?"=w309) -> (w306:cluster{"判断完成":bool, "不合格?":bool})
                        n345 = global write "全局 1.vi" "拨钮右左力检"(w306) -> ()
                      }
                      frame #2 {
                        n346 = Select(t=u32 0, s=w312, f=u32 16711680) -> (s? t:f=w311:u32)
                        n347 = property on="F拨钮右左" class="Str"("Text.TextColor"=w311, "Text.Text"=w310) -> ()  [unwired: 2 in, 2 out]
                      }
                    }
                  }
                }
                n348 = case shown="真" w283 {
                  tunnel: w287 -> [_ w316]
                  frame False {
                  }
                  frame True {
                    "拨钮右左" <- w316
                  }
                }
                n349 = case shown="真" w282 {
                  frame False {
                  }
                  frame True {
                    n350 = local write "选项卡控件"(T1."拨钮右->左" ("选项卡控件")) -> ()
                  }
                }
              }
              frame #4 {
                n351 = Unbundle By Name(w326) -> ("空动作"=w320:bool)
                n352 = Unbundle By Name(w325) -> ("拨钮上下"=w321:bool)
                n353 = global read "全局 1.vi" "拨钮上下Pr"() -> (w319:T5)
                n354 = property on="拨钮上下" class="WFChart (严格)"() -> ("History Data"=w323:sgl[])  [unwired: 2 in, 2 out]
                n355 = call "显示曲线.vi"("力觉参数"=w319, "力数组"=w327) -> ("力值"=w324:sgl)  [unwired: 1 in]
                n356 = call "处理信号.vi"("动作"=w321, "空动作"=w320) -> ("切换"=w318:bool, "显示曲线"=w317:bool, "判断"=w322:bool)  [unwired: 7 in]
                n357 = case shown="真" w322 {
                  tunnel: w323 -> [_ w333]
                  tunnel: w319 -> [_ w332]
                  frame False {
                  }
                  frame True {
                    n358 = Unbundle By Name(w332) -> ("上限"=w331:sgl, "下限"=w330:sgl, "起点"=w329:dbl, "终点"=w328:dbl)
                    n359 = call "曲线处理.vi"("上限"=w331, "下限"=w330, "起点"=w329, "终点"=w328, "历史数据"=w333) -> ("值显示"=w334:string, "曲线数组"=w336:sgl[], "范围内?"=w335:bool)  [unwired: 2 in, 1 out]
                    n360 = stacked-sequence {
                      tunnel: w336 -> [w341 _ _]
                      tunnel: w335 -> [_ w344 w349]
                      tunnel: w334 -> [_ _ w347]
                      frame #0 {
                        n361 = Array Size(array=w341) -> (size(s)=w340:i32)
                        n362 = To Double Precision Float(number=w340) -> (double precision float=w339:dbl)
                        n363 = Decrement(x=w339) -> (x-1=w338:dbl)
                        n364 = property on="拨钮上下" class="WFChart (严格)"("History Data"=w341, "XScale.Maximum"=w338, "XScale.Minimum"=0.0 ("X标尺.范围:最小值")) -> ()  [unwired: 2 in, 2 out]
                      }
                      frame #1 {
                        n365 = global read "全局 1.vi" "拨钮上下力检"() -> (w342:cluster{"判断完成":bool, "不合格?":bool})
                        n366 = Not(x=w344) -> (.not. x?=w346:bool)
                        n367 = Bundle By Name(cluster=w342, "判断完成"=TRUE, "不合格?"=w346) -> (w343:cluster{"判断完成":bool, "不合格?":bool})
                        n368 = global write "全局 1.vi" "拨钮上下力检"(w343) -> ()
                      }
                      frame #2 {
                        n369 = Select(t=u32 0, s=w349, f=u32 16711680) -> (s? t:f=w348:u32)
                        n370 = property on="F拨钮上下" class="Str"("Text.TextColor"=w348, "Text.Text"=w347) -> ()  [unwired: 2 in, 2 out]
                      }
                    }
                  }
                }
                n371 = case shown="真" w317 {
                  tunnel: w324 -> [_ w353]
                  frame False {
                  }
                  frame True {
                    "拨钮上下" <- w353
                  }
                }
                n372 = case shown="真" w318 {
                  frame False {
                  }
                  frame True {
                    n373 = local write "选项卡控件"(T1."拨钮上->下" ("选项卡控件")) -> ()
                  }
                }
              }
              frame #5 {
                n374 = Unbundle By Name(w363) -> ("空动作"=w358:bool)
                n375 = Unbundle By Name(w362) -> ("拨钮下上"=w359:bool)
                n376 = global read "全局 1.vi" "拨钮下上Pr"() -> (w354:T5)
                n377 = property on="拨钮下上" class="WFChart (严格)"() -> ("History Data"=w360:sgl[])  [unwired: 2 in, 2 out]
                n378 = call "处理信号.vi"("动作"=w359, "空动作"=w358) -> ("切换"=w356:bool, "显示曲线"=w357:bool, "判断"=w355:bool)  [unwired: 7 in]
                n379 = call "显示曲线.vi"("力觉参数"=w354, "力数组"=w364) -> ("力值"=w361:sgl)  [unwired: 1 in]
                n380 = case shown="真" w355 {
                  tunnel: w360 -> [_ w370]
                  tunnel: w354 -> [_ w369]
                  frame False {
                  }
                  frame True {
                    n381 = Unbundle By Name(w369) -> ("上限"=w368:sgl, "下限"=w367:sgl, "起点"=w366:dbl, "终点"=w365:dbl)
                    n382 = call "曲线处理.vi"("上限"=w368, "下限"=w367, "起点"=w366, "终点"=w365, "历史数据"=w370) -> ("值显示"=w371:string, "曲线数组"=w373:sgl[], "范围内?"=w372:bool)  [unwired: 2 in, 1 out]
                    n383 = stacked-sequence {
                      tunnel: w373 -> [w378 _ _]
                      tunnel: w372 -> [_ w381 w387]
                      tunnel: w371 -> [_ _ w385]
                      frame #0 {
                        n384 = Array Size(array=w378) -> (size(s)=w377:i32)
                        n385 = To Double Precision Float(number=w377) -> (double precision float=w376:dbl)
                        n386 = Decrement(x=w376) -> (x-1=w375:dbl)
                        n387 = property on="拨钮下上" class="WFChart (严格)"("History Data"=w378, "XScale.Maximum"=w375, "XScale.Minimum"=0.0 ("X标尺.范围:最小值")) -> ()  [unwired: 2 in, 2 out]
                      }
                      frame #1 {
                        n388 = global read "全局 1.vi" "拨钮下上力检"() -> (w380:cluster{"判断完成":bool, "不合格?":bool})
                        n389 = Not(x=w381) -> (.not. x?=w383:bool)
                        n390 = Bundle By Name(cluster=w380, "判断完成"=TRUE, "不合格?"=w383) -> (w379:cluster{"判断完成":bool, "不合格?":bool})
                        n391 = global write "全局 1.vi" "拨钮下上力检"(w379) -> ()
                      }
                      frame #2 {
                        n392 = Select(t=u32 0, s=w387, f=u32 16711680) -> (s? t:f=w386:u32)
                        n393 = property on="F拨钮下上" class="Str"("Text.TextColor"=w386, "Text.Text"=w385) -> ()  [unwired: 2 in, 2 out]
                      }
                    }
                  }
                }
                n394 = case shown="真" w357 {
                  tunnel: w361 -> [_ w390]
                  frame False {
                  }
                  frame True {
                    "拨钮下上" <- w390
                  }
                }
                n395 = case shown="真" w356 {
                  frame False {
                  }
                  frame True {
                    n396 = local write "选项卡控件"(T1."拨钮下->上" ("选项卡控件")) -> ()
                  }
                }
              }
              frame #6 {
                n397 = call "BuildSlaveRWr.vi"() -> ("RWr"=w391:i16[][])  [unwired: 1 in]
                n398 = call "BuildRX.vi"() -> ("RX"=w392:bool[][])  [unwired: 6 in]
              }
            }
            n399 = call "BuildResPDU.vi"("从站IP"=w138, "Node RX"=w126, "Node RWr"=w125, "占用站数"=w136, "主站信息"=w132) -> ("输出字符串"=w140:string, "主站IP"=w139:u32)  [unwired: 5 in]
            n400 = UDP Write(address=w139, port or service name=w142, connection ID=w144, data in=w140, 8:w146, 9:w133) -> (error out=w145:errorcluster, 3:w143:refnum<k16>)
          }
          frame Error {
            n401 = Unbundle By Name(w395) -> ("code"=w396:i32)
            n402 = case shown="56" w396 {
              tunnel: [w397 w398] -> w394
              tunnel: w395 -> [w397 _]
              frame Default {
              }
              frame 56 {
                w398 = errorcluster {"status"=FALSE, "code"=0, "source"=""}  # 无错误
              }
            }
          }
        }
        n403 = global read "全局 1.vi" "Exit"() -> (w112:bool)
        n404 = Wait (ms)(milliseconds to wait=u32 8 ("等待时间（毫秒）")) -> ()  [unwired: 1 out]
        n405 = Or(x=w112, y=w113) -> (x .or. y?=w120:bool)
      }
      n406 = UDP Close(connection ID=w108, 8:w106) -> ()  [unwired: 2 out]
    }
  }
  n407 = And(x=w4, y=TRUE) -> (x .and. y?=w3:bool)
  n408 = case shown="真" w3 {
    frame False {
    }
    frame True {
      n409 = invoke class="VI" method="FP.Close"() -> (reference out=w667:refnum<vi>, error out=w668:errorcluster)  [unwired: 3 in, 1 out]
      n410 = Close Reference(reference=w667, error in (no error)=w668) -> ()  [unwired: 1 out]
    }
  }
